vi "Configure Serial Bus (Flexray - Trigger).vi"(0 "VISA resource name":refnum<visa-resource-name>, 5 "Serial Bus Name (1: Serial Bus 1)":i32(ring)=1 items=["Serial Bus 1"=1, "Serial Bus 2"=2], 9 "Trigger Mode (0: Frame)":i32(ring) items=["Frame", "Error", "Event"], 11 "error in (no error)":errorcluster) -> (4 "VISA resource name out":refnum<visa-resource-name>, 15 "error out":errorcluster)   [LabVIEW 2010, in "Agilent 2000 3000 X-Series.lvlib"]
doc: "Configures the trigger type of FlexRay bus."
uses:
  <instrlib>/Agilent 2000 3000 X-Series/Agilent 2000 3000 X-Series.lvlib
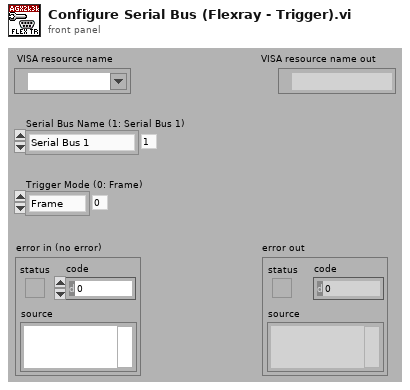
[diagram p1: front panel]
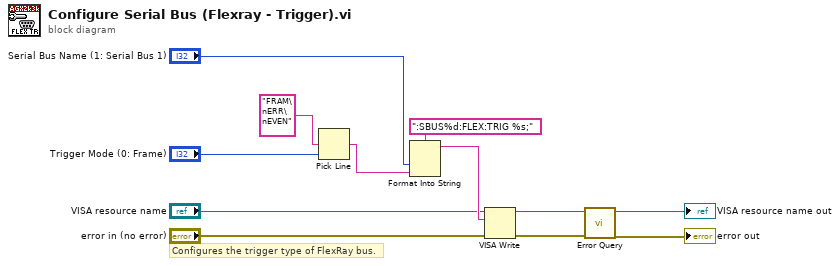
[diagram p0: block diagram]
diagram:
  # "Configures the trigger type of FlexRay bus."
  n1 = Pick Line(multi-line string="FRAM\nERR\nEVEN", line index="Trigger Mode (0: Frame)") -> (output string=w8:string)  [unwired: 1 out]
  n2 = Format Into String(format string=":SBUS%d:FLEX:TRIG %s;", "Serial Bus Name (1: Serial Bus 1)", w8) -> (resulting string=w7:string)  [unwired: 2 in, 1 out]
  n3 = VISA Write(VISA resource name="VISA resource name", write buffer=w7, error in (no error)="error in (no error)") -> (VISA resource name out=w4:refnum<visa-resource-name>, error out=w3:errorcluster)  [unwired: 1 out]
  n4 = call <instrlib>:"Error Query.vi"("error in (no error)"=w3, "VISA resource name"=w4) -> ("error out"=→"error out":errorcluster, "VISA resource name out"=→"VISA resource name out":refnum<visa-resource-name>)  [unwired: 8 out]
